vi "Dequeue Timed Out.vi"(4 "priority in":i32, 6 "timed out?":bool, 7 "Wait Prior":refnum<queue>, 8 "error in (no error)":errorcluster, 9 "element in":refnum<class "Message.lvclass">, 10 "wait queue":refnum<queue>, 11 "priority queue":refnum<data-value>) -> (0 "error out":errorcluster, 1 "priority out":i32, 2 "element out":refnum<class "Message.lvclass">, 3 "really timed out?":bool)   [LabVIEW 2013, in "Actor Framework.lvlib" / "Message Priority Queue.lvclass"]
uses:
  <vilib>/ActorFramework/Message Priority Queue/Message Priority Queue.lvclass
  <vilib>/ActorFramework/Message Priority Queue/DVR Contents.ctl
  <vilib>/ActorFramework/Message/Message.lvclass
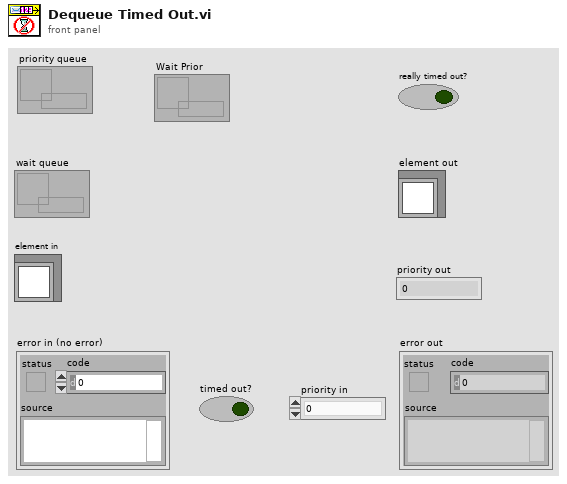
[diagram p1: front panel]
types:
  T1 = typedef "Actor Framework.lvlib/Message Priority Queue.lvclass/DVR Contents.ctl" = cluster{"# Waiting":u32, "Buffers":refnum<queue>[], "Wait Msg":refnum<queue>, "Wait Prior":refnum<queue>}
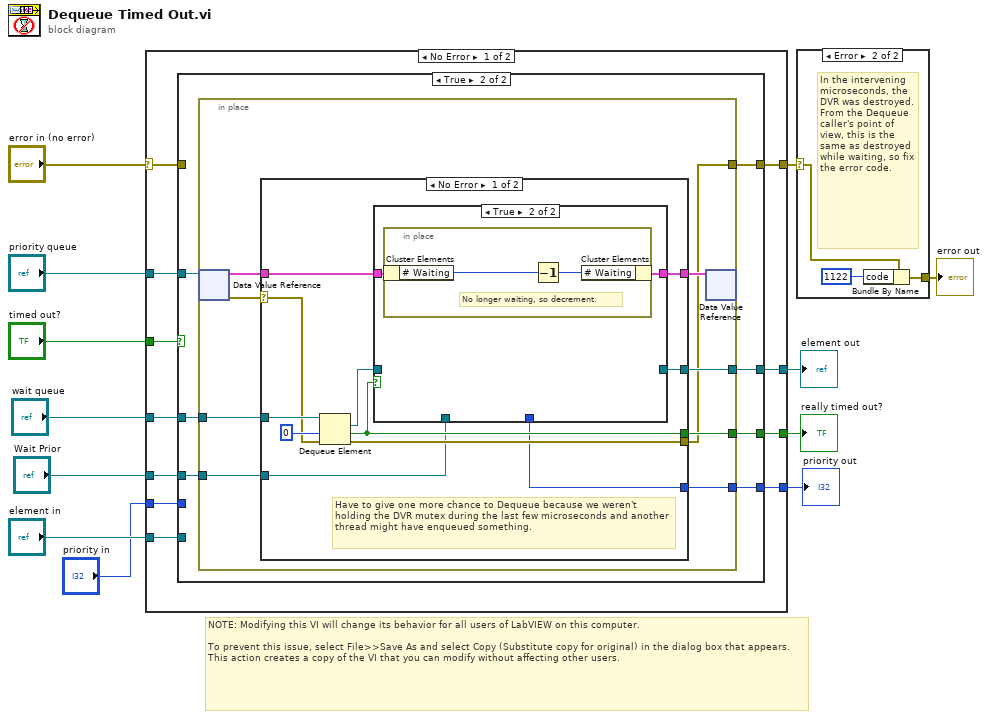
[diagram p0: block diagram]
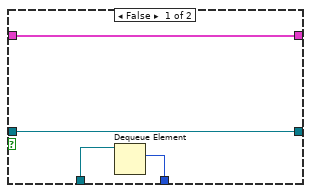
[diagram p4: hidden frame]
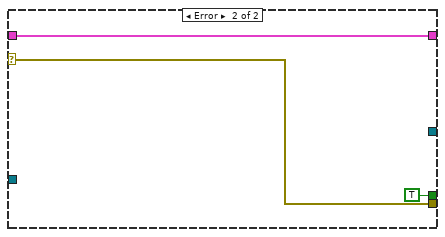
[diagram p5: hidden frame]
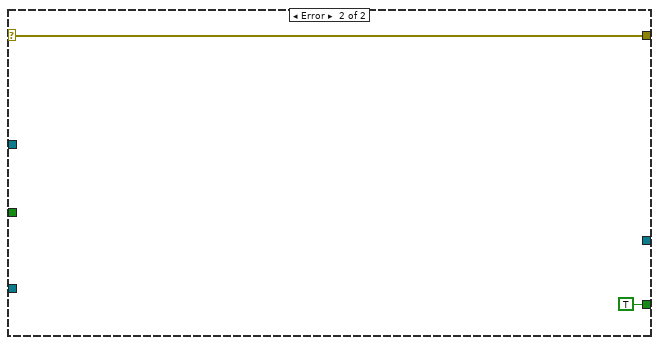
[diagram p6: hidden frame]
diagram:
  # "NOTE: Modifying this VI will change its behavior for all users of LabVIEW on this computer.\n\nTo prevent this issue, select File>>Save As and select Copy (Substitute copy for original) in the dialog box that appears. This action creates a copy of the VI that you can modify without affecting other users."
  n1 = case shown="No Error" "error in (no error)" {
    selector: "error in (no error)" -> [w16 w67]
    tunnel: "priority queue" -> [w23 _]
    tunnel: [w22 _] -> w11
    tunnel: "element in" -> [w21 _]
    tunnel: "wait queue" -> [w20 _]
    tunnel: [w19 TRUE ("timed out?")] -> w9
    tunnel: "timed out?" -> [w18 _]
    tunnel: [w17 w67] -> w6
    tunnel: "Wait Prior" -> [w15 _]
    tunnel: [w14 _] -> w2
    tunnel: "priority in" -> [w13 _]
    frame No Error {
      n2 = case shown="True" w18 {
        selector: w18 -> [w27 _]
        tunnel: [w27 w32] -> w19
        tunnel: w20 -> [_ w33]
        tunnel: w21 -> [w26 _]
        tunnel: [w26 w31] -> w22
        tunnel: w23 -> [_ w34]
        tunnel: [w25 w30] -> w17
        tunnel: w16 -> [w25 _]
        tunnel: w15 -> [_ w29]
        tunnel: [w24 w28] -> w14
        tunnel: w13 -> [w24 _]
        frame False {
        }
        frame True {
          n3 = in-place {
            in-place-border: w33 -> [w43]
            in-place-border: [w42] -> w32
            in-place-border: [w39] -> w31
            in-place-border: [w37] -> w30
            in-place-border: w29 -> [w36]
            in-place-border: [w35] -> w28
            n4 = in-place-dvr #1(w34) -> (w40:T1, w38:errorcluster)
            n5 = case shown="No Error" w38 {
              selector: w38 -> [w47 w63]
              tunnel: w43 -> [w54 _]
              tunnel: [w52 TRUE ("timed out?")] -> w42
              tunnel: [w51 w65] -> w41
              tunnel: w40 -> [w50 w65]
              tunnel: [w49 _] -> w39
              tunnel: [w46 w63] -> w37
              tunnel: w36 -> [w45 _]
              tunnel: [w44 _] -> w35
              frame No Error {
                # "Have to give one more chance to Dequeue because we weren't holding the DVR mutex during the last few microseconds and another thread might have enqueued something."
                n6 = Dequeue Element(queue=w54, timeout in ms (-1)=0, error in (no error)=w47) -> (element=w48:refnum<class "Message.lvclass">, timed out?=w52:bool, error out=w46:errorcluster)  [unwired: 1 out]
                n7 = case shown="True" w52 {
                  tunnel: [w58 w59] -> w51
                  tunnel: w50 -> [w58 w60]
                  tunnel: [w57 _] -> w49
                  tunnel: w48 -> [w57 _]
                  tunnel: w45 -> [w56 _]
                  tunnel: [w55 _] -> w44
                  frame False {
                    n8 = Dequeue Element(queue=w56) -> (element=w55:i32)  [unwired: 2 in, 3 out]
                  }
                  frame True {
                    n9 = in-place {
                      # "No longer waiting, so decrement."
                      n10 = in-place-cluster #2(w60) -> ("# Waiting"=w62:u32)
                      n11 = Decrement(x=w62) -> (x-1=w61:u32)
                      n12 = in-place-cluster #2("# Waiting"=w61) -> (w59:T1)
                    }
                  }
                }
              }
              frame Error {
              }
            }
            n13 = in-place-dvr #1(w41) -> ()  [unwired: 2 out]
          }
        }
      }
    }
    frame Error {
    }
  }
  "element out" <- w11
  "really timed out?" <- w9
  "priority out" <- w2
  n14 = case shown="Error" w6 {
    selector: w6 -> [w68 w69]
    tunnel: [w68 w70] -> w7
    frame No Error {
    }
    frame Error {
      # "In the intervening microseconds, the DVR was destroyed. From the Dequeue caller's point of view, this is the same as destroyed while waiting, so fix the error code."
      n15 = Bundle By Name(cluster=w69, "code"=1122) -> (w70:errorcluster)
    }
  }
  "error out" <- w7
